vi "op_num_l0.vi"() -> ()   [LabVIEW 2009]
panel:
  in  "stop":bool
  out "led":bool
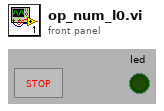
[diagram p1: front panel]
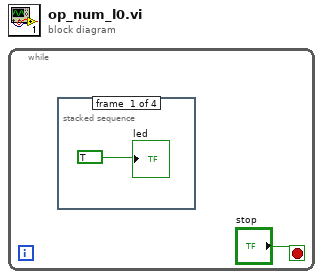
[diagram p0: block diagram]
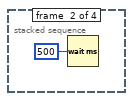
[diagram p2: hidden frame]
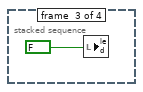
[diagram p3: hidden frame]
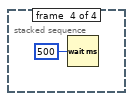
[diagram p4: hidden frame]
diagram:
  n1 = while {
    stop <- "stop" stop-if-true
    n2 = stacked-sequence {
      frame #0 {
        "led" <- TRUE ("led")
      }
      frame #1 {
        n3 = Wait (ms)(milliseconds to wait=u32 500) -> ()  [unwired: 1 out]
      }
      frame #2 {
        n4 = local write "led"(FALSE ("led")) -> ()
      }
      frame #3 {
        n5 = Wait (ms)(milliseconds to wait=u32 500) -> ()  [unwired: 1 out]
      }
    }
  }
